vi "ContDecodeProgramIterations.vi"(11 "Continuous Program in":string[][](array[string])) -> (3 "Continuous Program out":string[][](array[string]))   [LabVIEW 2018]
uses:
  <vilib>/regexp/Match Regular Expression.xnode
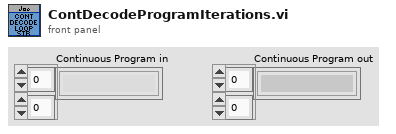
[diagram p1: front panel]
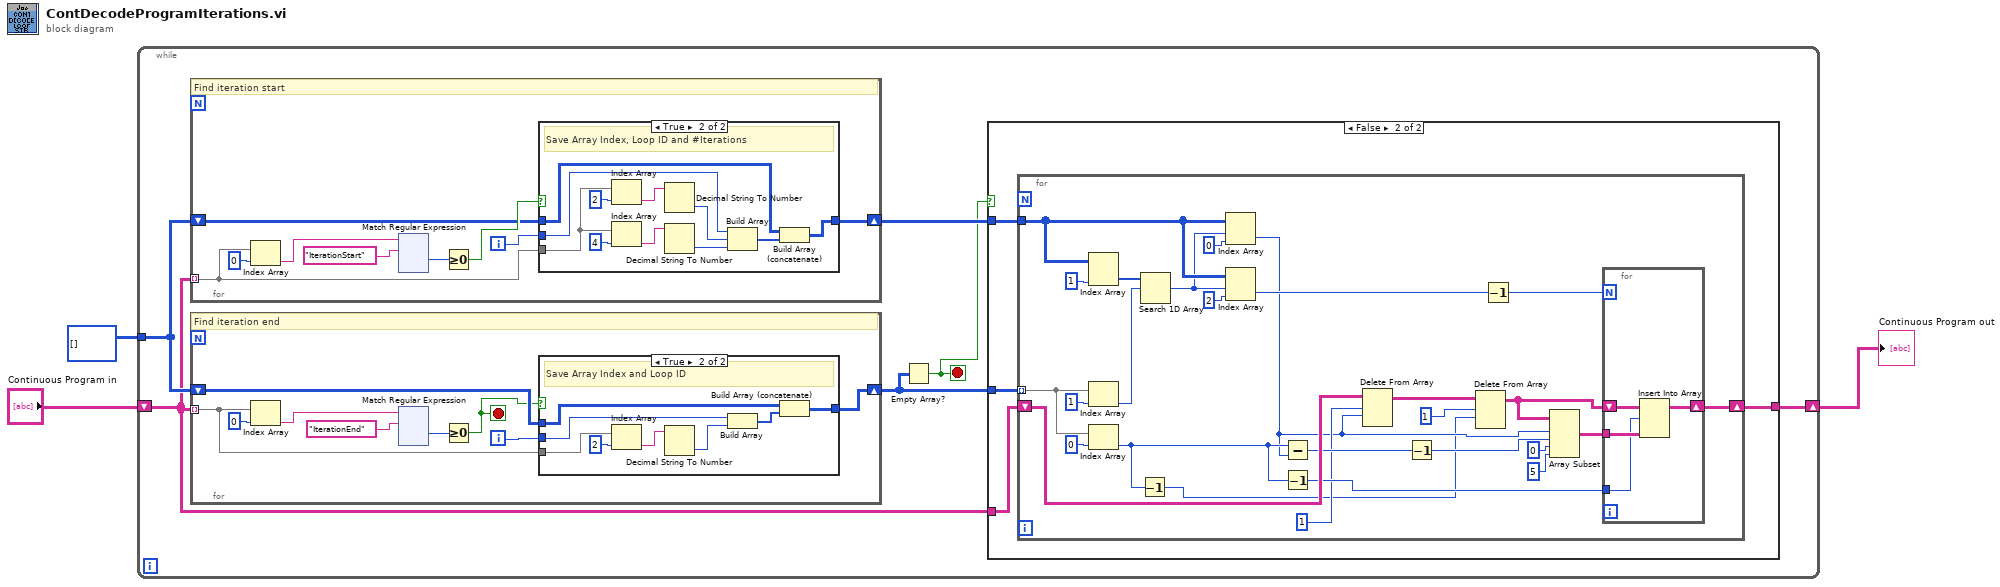
[diagram p0: block diagram]
diagram:
  n1 = while {
    tunnel: i32[][] [] -> [w9]
    shift-right: [w6] -> w3
    shift-left: "Continuous Program in" -> [w7]
    stop <- w4 stop-if-true
    n2 = for {
      shift-right: [w183] -> w8
      shift-left: w9 -> [w182]
      tunnel: w7 -> [w179] mode=indexing
      i -> [w178]
      # "Find iteration start"
      n3 = Index Array(array=w179, index=0 ("disabled index (col)")) -> (element=w181:string)
      n4 = xnode "Match Regular Expression"("input string"=w181, "regular expression"="IterationStart" ("element")) -> ("offset past match"=w185:i32)  [unwired: 4 in, 4 out]
      n5 = Greater Or Equal To 0?(x=w185) -> (x >= 0?=w184:bool)
      n6 = case shown="True" w184 {
        tunnel: [w187 w198] -> w183
        tunnel: w182 -> [w187 w197]
        tunnel: w179 -> [_ w190]
        tunnel: w178 -> [_ w196]
        frame False {
        }
        frame True {
          # "Save Array Index, Loop ID and #Iterations"
          n7 = Index Array(array=w190, index=2 ("disabled index (col)")) -> (element=w193:string)
          n8 = Index Array(array=w190, index=4 ("disabled index (col)")) -> (element=w191:string)
          n9 = Decimal String To Number(string=w193) -> (number=w189:i32)  [unwired: 2 in, 1 out]
          n10 = Decimal String To Number(string=w191) -> (number=w188:i32)  [unwired: 2 in, 1 out]
          n11 = Build Array(w196, w189, w188) -> (w195:i32[])
          n12 = Build Array (concatenate)(w197, w195) -> (w198:i32[][])
        }
      }
    }
    n13 = for {
      shift-right: [w52] -> w5
      shift-left: w9 -> [w51]
      tunnel: w7 -> [w48] mode=indexing
      i -> [w47]
      stop <- w46 stop-if-true
      # "Find iteration end"
      n14 = Index Array(array=w48, index=0 ("disabled index (col)")) -> (element=w50:string)
      n15 = xnode "Match Regular Expression"("input string"=w50, "regular expression"="IterationEnd" ("element")) -> ("offset past match"=w53:i32)  [unwired: 4 in, 4 out]
      n16 = Greater Or Equal To 0?(x=w53) -> (x >= 0?=w46:bool)
      n17 = case shown="True" w46 {
        tunnel: [w55 w63] -> w52
        tunnel: w51 -> [w55 w62]
        tunnel: w48 -> [_ w60]
        tunnel: w47 -> [_ w57]
        frame False {
        }
        frame True {
          # "Save Array Index and Loop ID"
          n18 = Index Array(array=w60, index=2 ("disabled index (col)")) -> (element=w59:string)
          n19 = Decimal String To Number(string=w59) -> (number=w58:i32)  [unwired: 2 in, 1 out]
          n20 = Build Array(w57, w58) -> (w56:i32[])
          n21 = Build Array (concatenate)(w62, w56) -> (w63:i32[][])
        }
      }
    }
    n22 = Empty Array?(array=w5) -> (empty?=w4:bool)
    n23 = case shown="False" w4 {
      tunnel: w8 -> [_ w14]
      tunnel: w7 -> [w10 w13]
      tunnel: [w10 w12] -> w6
      tunnel: w5 -> [_ w11]
      frame True {
      }
      frame False {
        n24 = for {
          tunnel: w14 -> [w18]
          tunnel: w11 -> [w29] mode=indexing
          shift-right: [w27] -> w12
          shift-left: w13 -> [w41]
          n25 = Index Array(array=w18, index (col)=1 ("index")) -> (element=w26:i32[])  [unwired: 1 in]
          n26 = Index Array(array=w29, index=1 ("disabled index (col)")) -> (element=w24:i32)
          n27 = Index Array(array=w29, index=0 ("disabled index (col)")) -> (element=w30:i32)
          n28 = Decrement(x=w30) -> (x-1=w19:i32)
          n29 = Search 1D Array(1D array=w26, element=w24) -> (index of element=w16:i32)  [unwired: 1 in]
          n30 = Index Array(array=w18, index (row)=w16, index (col)=0 ("index")) -> (element=w20:i32)
          n31 = Index Array(array=w18, index (row)=w16, index (col)=2 ("disabled index (col)")) -> (element=w28:i32)
          n32 = Subtract(x=w30, y=w20) -> (x-y=w40:i32)
          n33 = Decrement(x=w30) -> (x-1=w35:i32)
          n34 = Delete From Array(array=w41, length=1, index (row)=w20) -> (array with subset deleted=w32:string[][])  [unwired: 1 in, 1 out]
          n35 = Decrement(x=w40) -> (x-1=w39:i32)
          n36 = Delete From Array(array=w32, length=1, index (row)=w19) -> (array with subset deleted=w31:string[][])  [unwired: 1 in, 1 out]
          n37 = Decrement(x=w28) -> (x-1=w15:i32)
          n38 = Array Subset(array=w31, index (row)=w20, length (row)=w39, index (col)=0 ("index"), length (col)=5 ("length")) -> (w36:string[][])
          n39 = for {
            N: w15 -> [_]
            tunnel: w36 -> [w44]
            tunnel: w35 -> [w43]
            shift-right: [w42] -> w27
            shift-left: w31 -> [w45]
            n40 = Insert Into Array(array=w45, index (row)=w43, new element=w44) -> (w42:string[][])  [unwired: 1 in]
          }
        }
      }
    }
  }
  "Continuous Program out" <- w3
